vi "Get VI Inputs and Outputs.vi"   [LabVIEW 2016, in "SLL Application.lvlib"]
uses:
  SLL Application.lvlib
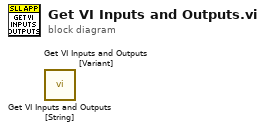
[diagram p0: block diagram]
diagram:
  n1 = call "Get VI Inputs and Outputs [String].vi"() -> ()  [unwired: 8 in, 4 out]
  n2 = call "Get VI Inputs and Outputs [Variant].vi"() -> ()  [unwired: 8 in, 4 out]
